vi "Write Result Msg.vi"(10 "Inference.lvlib:Result Msg.lvclass":refnum<class "Result Msg.lvclass">, 11 "Inference in":refnum<class "Inference.lvclass">) -> (3 "Inference out":refnum<class "Inference.lvclass">)   [LabVIEW 2019, in "Inference.lvlib" / "Inference.lvclass"]
uses:
  Inference.lvclass
  Inference Messages/Result Msg/Result Msg.lvclass
  Inference.lvclass/Inference.ctl
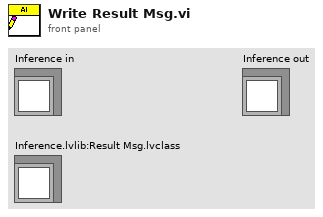
[diagram p1: front panel]
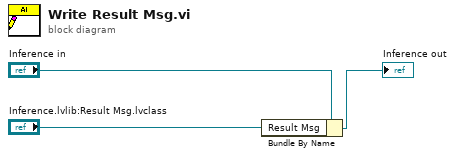
[diagram p0: block diagram]
diagram:
  n1 = Bundle By Name(cluster="Inference in", "Result Msg"="Inference.lvlib:Result Msg.lvclass") -> (→"Inference out":refnum<class "Inference.lvclass">)
